vi "Function_Wizard.vi"(6 "Input":dbl[][](array[numeric]), 7 "Device References":refnum<vi>[](array[refnum]), 8 "Device properties":cluster{"Number of axes":i32}[](array[cluster]), 9 "Device parameters":variant[](array[variant]), 10 "Device order":i32[](array[numeric])=[0, 1], 11 "Device description":string[][](array[string])) -> (3 "Output":dbl[][](array[numeric]))   [LabVIEW 2015]
uses:
  <vilib>/gmath/NI_Gmath.lvlib
panel:
  in  "Cancel Button":bool
  in  "OK Button":bool
  in  "Ordering":u16(ring) items=["Raster", "Serpentine"]
  in  "Expression":string
  in  "Scan pattern":u16(ring) items=["Linear", "Exponential", "Logarithmic", "Quadratic", "Custom"]
  in  "Parameter table":string[][](table)
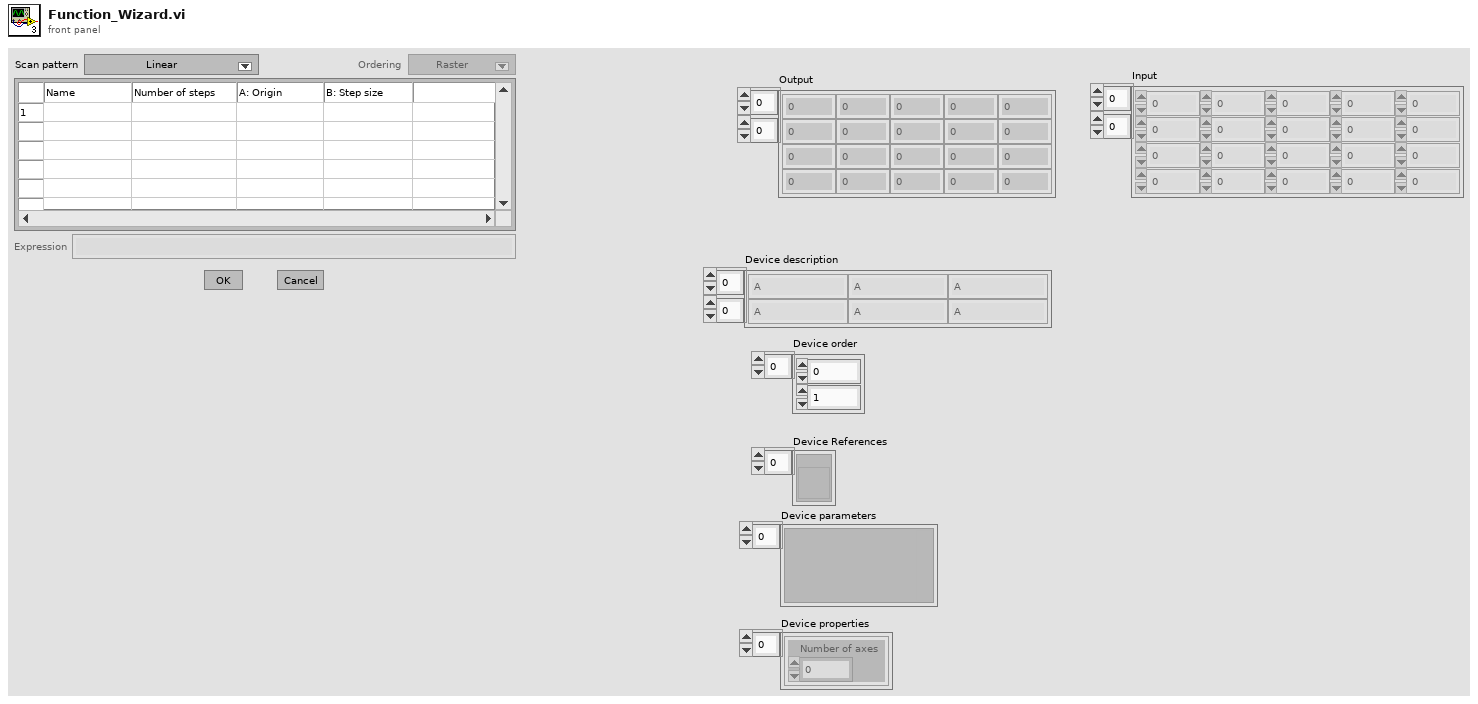
[diagram p1: front panel]
types:
  T1 = enum8{"Enabled", "Disabled", "Disabled and Grayed Out"}
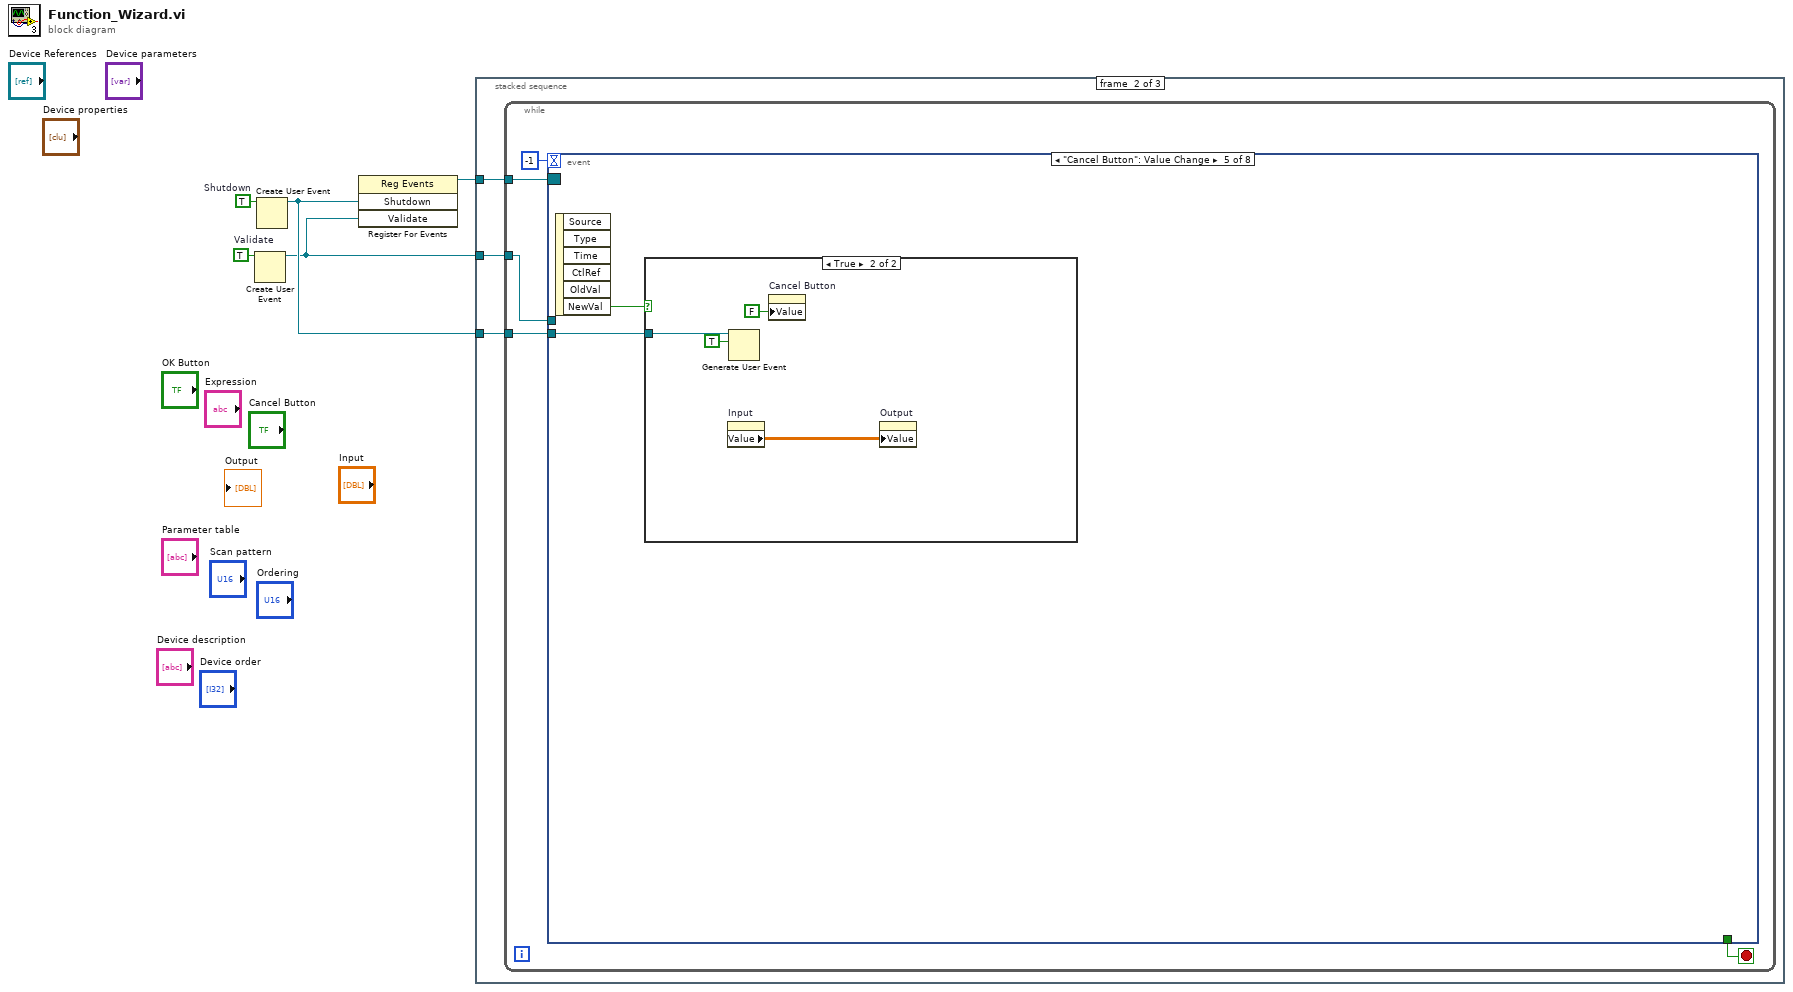
[diagram p0: block diagram]
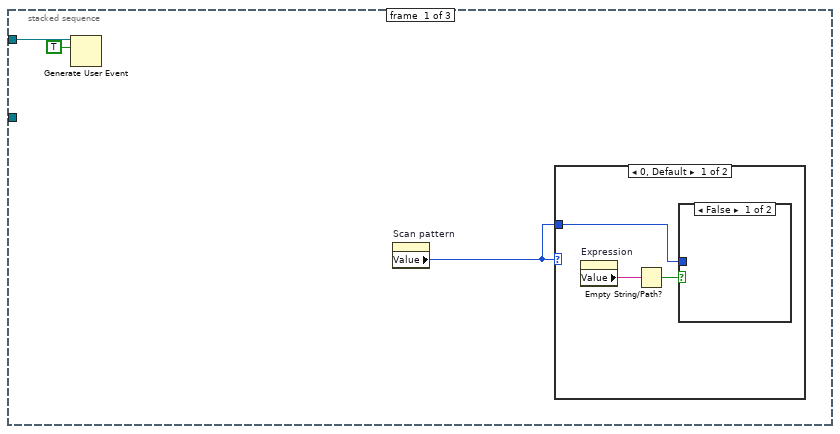
[diagram p2: hidden frame]
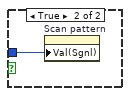
[diagram p3: hidden frame]
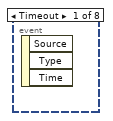
[diagram p5: hidden frame]
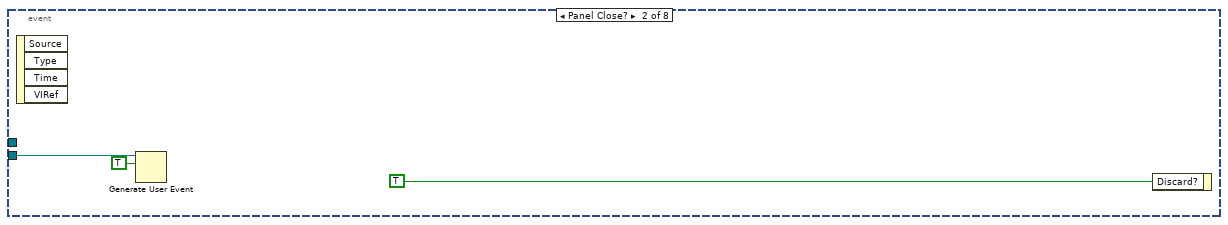
[diagram p6: hidden frame]
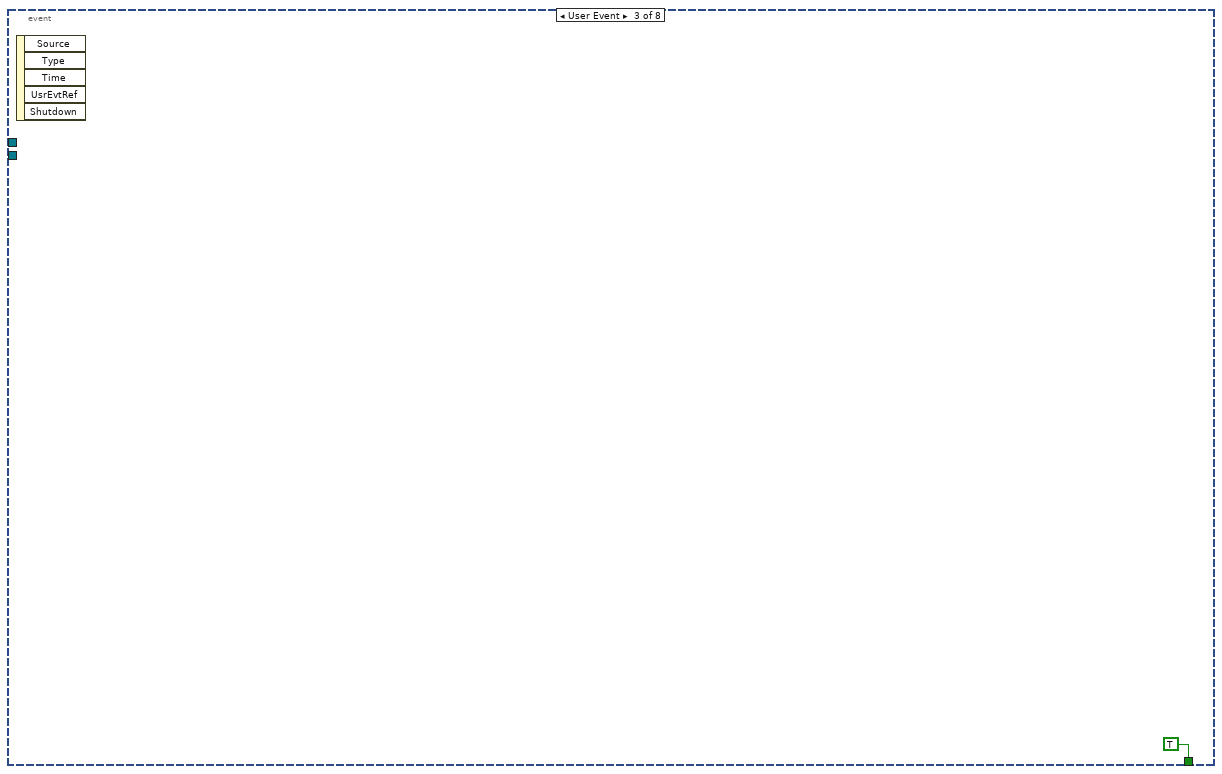
[diagram p7: hidden frame]
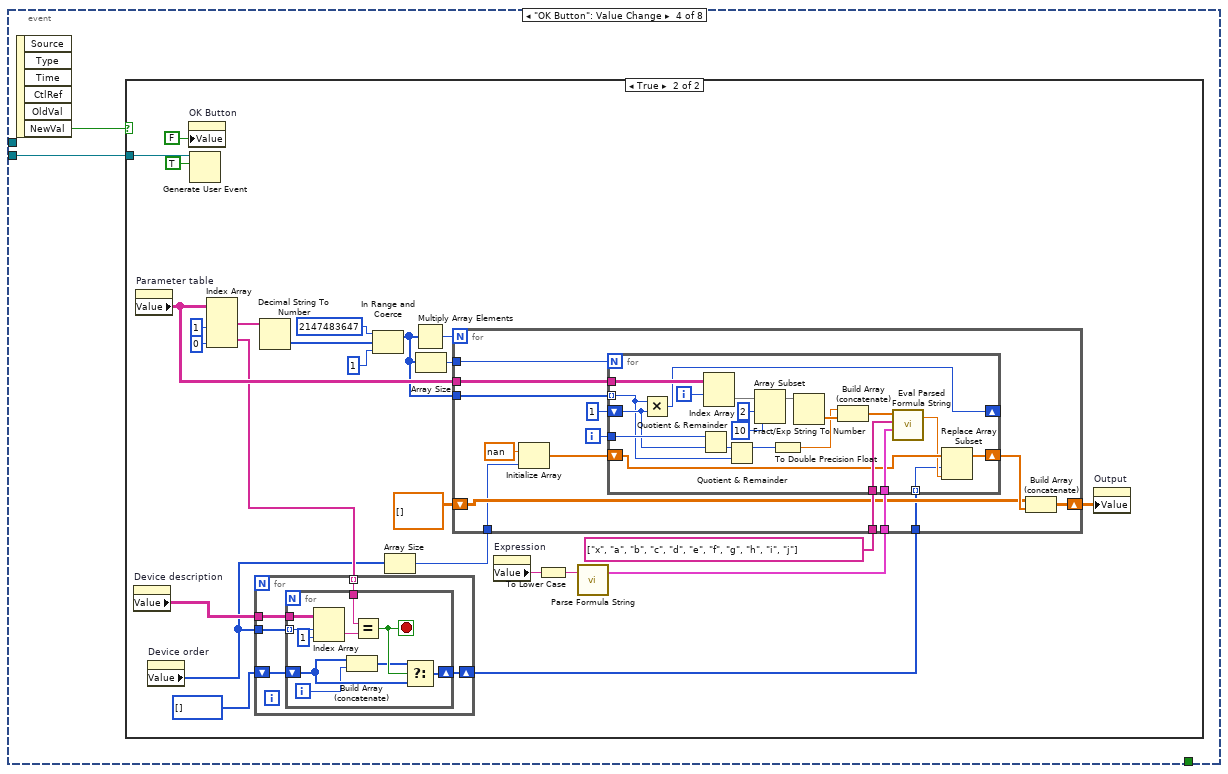
[diagram p8: hidden frame]
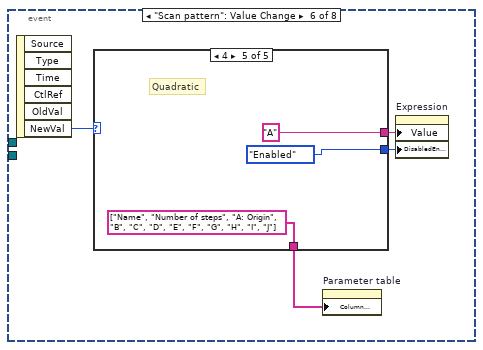
[diagram p11: hidden frame]
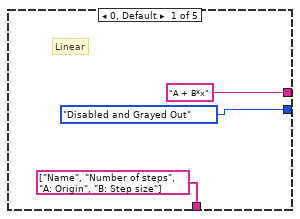
[diagram p12: hidden frame]
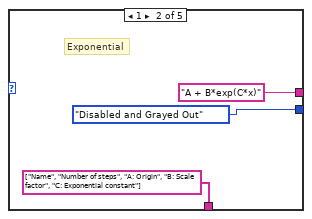
[diagram p13: hidden frame]
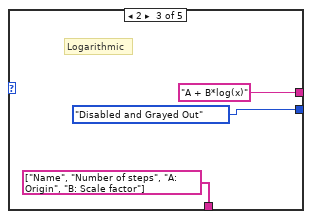
[diagram p14: hidden frame]
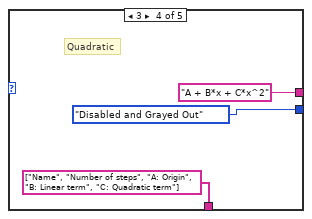
[diagram p15: hidden frame]
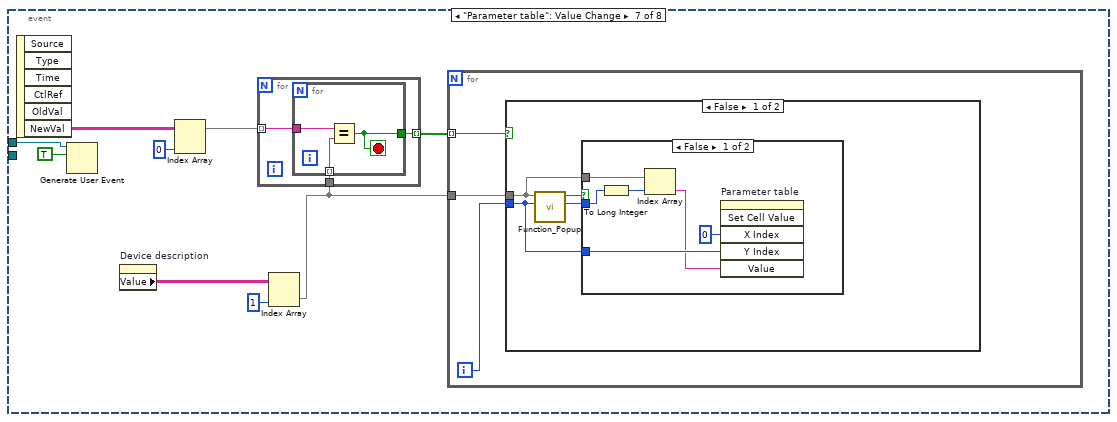
[diagram p16: hidden frame]
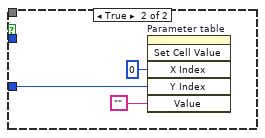
[diagram p17: hidden frame]
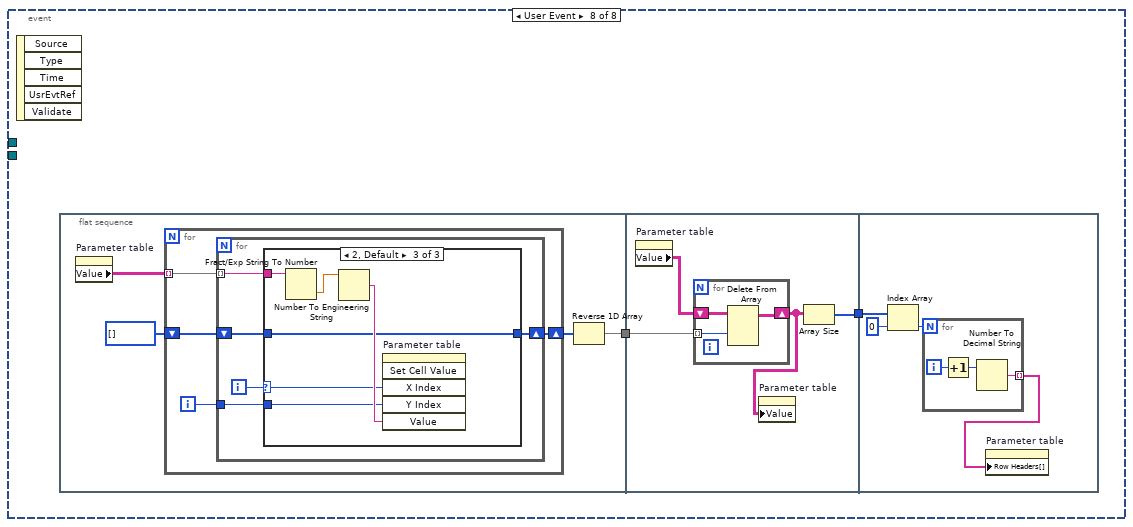
[diagram p19: hidden frame]
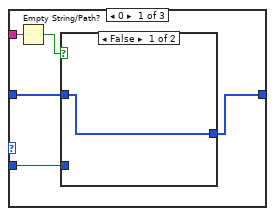
[diagram p20: hidden frame]
diagram:
  w2 = TRUE  # Validate
  w4 = TRUE  # Shutdown
  n1 = Create User Event(user event datatype=w2) -> (user event=w1:refnum<user-event>)  [unwired: 1 in, 1 out]
  n2 = Create User Event(user event datatype=w4) -> (user event=w3:refnum<user-event>)  [unwired: 1 in, 1 out]
  n3 = register-events(w3, w1) -> (reference out=w5:refnum<event-registration>)  [unwired: 2 in, 1 out]
  n4 = stacked-sequence {
    tunnel: w5 -> [_ w15 _]
    tunnel: w3 -> [_ w14 w208]
    tunnel: w1 -> [w8 w13 w209]
    frame #0 {
      n5 = Generate User Event(user event=w8, event data cluster=TRUE ("event data")) -> ()  [unwired: 2 in, 2 out]
      n6 = property on="Scan pattern" class="Ring (strict)"() -> ("Value"=w6:u16)  [unwired: 2 in, 2 out]
      n7 = case shown="0, Default" w6 {
        tunnel: w6 -> [w9 _]
        frame 0, Default {
          n8 = property on="Expression" class="Str"() -> ("Value"=w11:string)  [unwired: 2 in, 2 out]
          n9 = Empty String/Path?(string/path=w11) -> (empty?=w10:bool)
          n10 = case shown="False" w10 {
            tunnel: w9 -> [_ w12]
            frame False {
            }
            frame True {
              n11 = property on="Scan pattern" class="Ring (strict)"("Val(Sgnl)"=w12) -> ()  [unwired: 2 in, 2 out]
            }
          }
        }
        frame 4 {
        }
      }
    }
    frame #1 {
      n12 = while {
        tunnel: w15 -> [w19]
        tunnel: w14 -> [w17]
        tunnel: w13 -> [w16]
        stop <- w18 stop-if-true
        n13 = event shown="[4] \"Cancel Button\": Value Change" {
          selector: w19 -> [_ _ _ _ _ _ _ _]
          dyn-events: _ -> [_ _ _ _ _ _ _ _]
          timeout: -1 -> [_ _ _ _ _ _ _ _]
          tunnel: [_ _ TRUE _ _ _ _ _] -> w18
          tunnel: w17 -> [_ w22 _ w26 w103 _ _ _]
          tunnel: w16 -> [_ _ _ _ _ _ w135 _]
          event Timeout {
            n14 = event-data() -> ()  [unwired: 1 in, 3 out]
          }
          event Panel Close? {
            n15 = event-data() -> ()  [unwired: 1 in, 4 out]
            n16 = Generate User Event(user event=w22, event data cluster=TRUE ("event data")) -> ()  [unwired: 2 in, 2 out]
            n17 = event-data("Discard?"=TRUE) -> ()  [unwired: 1 in, 1 out]
          }
          event User Event {
            n18 = event-data() -> ()  [unwired: 1 in, 5 out]
          }
          event "OK Button": Value Change {
            n19 = event-data() -> ("NewVal"=w25:bool)  [unwired: 1 in, 5 out]
            n20 = case shown="True" w25 {
              tunnel: w26 -> [_ w51]
              frame False {
              }
              frame True {
                n21 = property on="Device description" class="Arr (strict)"() -> ("Value"=w32:string[][])  [unwired: 2 in, 2 out]
                n22 = property on="Parameter table" class="Tbl (strict)"() -> ("Value"=w41:string[][])  [unwired: 2 in, 2 out]
                n23 = property on="Device order" class="Arr (strict)"() -> ("Value"=w27:i32[])  [unwired: 2 in, 2 out]
                n24 = property on="OK Button" class="Bool (strict)"("Value"=FALSE ("OK Button")) -> ()  [unwired: 2 in, 2 out]
                n25 = Generate User Event(user event=w51, event data cluster=TRUE ("event data")) -> ()  [unwired: 2 in, 2 out]
                n26 = Index Array(array=w41, index (col) #1=1 ("disabled index (col)"), index (col) #2=0 ("index (col)")) -> (element #1=w47:string[], element #2=w31:string[])  [unwired: 2 in]
                n27 = for {
                  tunnel: w32 -> [w56]
                  tunnel: w27 -> [w55]
                  tunnel: w31 -> [w54] mode=indexing
                  shift-right: [w52] -> w29
                  shift-left: i32[] [] -> [w53]
                  n28 = for {
                    tunnel: w56 -> [w66]
                    tunnel: w55 -> [w65] mode=indexing
                    tunnel: w54 -> [w63]
                    shift-right: [w61] -> w52
                    shift-left: w53 -> [w60]
                    i -> [w57]
                    stop <- w62 stop-if-true
                    n29 = Index Array(array=w66, index (row)=w65, index (col)=1 ("disabled index (col)")) -> (element=w58:string)
                    n30 = Build Array (concatenate)(w60, w57) -> (w59:i32[])
                    n31 = Equal?(x=w63, y=w58) -> (x = y?=w62:bool)
                    n32 = Select(t=w59, s=w62, f=w60) -> (s? t:f=w61:i32[])
                  }
                }
                n33 = Decimal String To Number(string=w47) -> (number=w46:i32[])  [unwired: 2 in, 1 out]
                n34 = In Range and Coerce(upper limit=2147483647, x=w46, lower limit=1) -> (coerced(x)=w38:i32[])  [unwired: 1 out]
                n35 = Array Size(array=w27) -> (size(s)=w28:i32)
                n36 = Multiply Array Elements(1:w38) -> (0:w44:i32)
                n37 = Array Size(array=w38) -> (size(s)=w43:i32)
                n38 = property on="Expression" class="Str"() -> ("Value"=w35:string)  [unwired: 2 in, 2 out]
                n39 = To Lower Case(string=w35) -> (all lower case string=w34:string)
                n40 = call <vilib>:"Parse Formula String.vi"("formula"=w34) -> ("Parsed Formula"=w40:cluster{"Table":i32[][], "Y Values":dbl[]})  [unwired: 1 in, 1 out]
                n41 = for {
                  N: w44 -> [_]
                  tunnel: w43 -> [w78]
                  tunnel: w41 -> [w80]
                  tunnel: w40 -> [w76]
                  tunnel: string[] ["x", "a", "b", "c", "d", "e", "f", "g", "h", "i", "j"] ("Variables") -> [w75]
                  tunnel: w38 -> [w70]
                  shift-right: [w71] -> w36
                  shift-left: dbl[][] [] -> [w72]
                  tunnel: w29 -> [w68]
                  tunnel: w28 -> [w67]
                  i -> [w74]
                  n42 = Initialize Array(nan ("element"), w67) -> (w79:dbl[])
                  n43 = for {
                    N: w78 -> [_]
                    tunnel: w80 -> [w101]
                    shift-right: [w89] -> w73
                    shift-left: w79 -> [w88]
                    tunnel: w76 -> [w97]
                    tunnel: w75 -> [w96]
                    tunnel: w74 -> [w85]
                    shift-right: [w92] -> _
                    shift-left: 1 -> [w83]
                    tunnel: w70 -> [w82] mode=indexing
                    tunnel: w68 -> [w81] mode=indexing
                    i -> [w86]
                    n44 = Multiply(x=w82, y=w83) -> (x*y=w92:i32)
                    n45 = Quotient & Remainder(x=w85, y=w83) -> (floor(x/y)=w84:i32)  [unwired: 1 out]
                    n46 = Index Array(array=w101, index (row)=w86) -> (element=w100:string[])  [unwired: 1 in]
                    n47 = Quotient & Remainder(x=w84, y=w82) -> (x-y*floor(x/y)=w91:i32)  [unwired: 1 out]
                    n48 = Array Subset(array=w100, index=2, length=10) -> (w99:string[])
                    n49 = To Double Precision Float(number=w91) -> (double precision float=w90:dbl)
                    n50 = Fract/Exp String To Number(string=w99) -> (number=w95:dbl[])  [unwired: 3 in, 1 out]
                    n51 = Build Array (concatenate)(w90, w95) -> (w94:dbl[])
                    n52 = call <vilib>:"Eval Parsed Formula String.vi"("Parsed Formula"=w97, "Variables"=w96, "X Values"=w94) -> ("y value"=w87:dbl)  [unwired: 1 in, 1 out]
                    n53 = Replace Array Subset(array=w88, new element=w87, index=w81) -> (w89:dbl[])
                  }
                  n54 = Build Array (concatenate)(w72, w73) -> (w71:dbl[][])
                }
                n55 = property on="Output" class="Arr (strict)"("Value"=w36) -> ()  [unwired: 2 in, 2 out]
              }
            }
          }
          event "Cancel Button": Value Change {
            n56 = event-data() -> ("NewVal"=w102:bool)  [unwired: 1 in, 5 out]
            n57 = case shown="True" w102 {
              tunnel: w103 -> [_ w107]
              frame False {
              }
              frame True {
                n58 = property on="Input" class="Arr (strict)"() -> ("Value"=w104:dbl[][])  [unwired: 2 in, 2 out]
                n59 = Generate User Event(user event=w107, event data cluster=TRUE ("event data")) -> ()  [unwired: 2 in, 2 out]
                n60 = property on="Cancel Button" class="Bool (strict)"("Value"=FALSE ("Cancel Button")) -> ()  [unwired: 2 in, 2 out]
                n61 = property on="Output" class="Arr (strict)"("Value"=w104) -> ()  [unwired: 2 in, 2 out]
              }
            }
          }
          event "Scan pattern": Value Change {
            n62 = event-data() -> ("NewVal"=w111:u16)  [unwired: 1 in, 5 out]
            n63 = case shown="4" w111 {
              tunnel: ["A + B*x" "A + B*exp(C*x)" "A + B*log(x)" "A + B*x + C*x^2" "A"] -> w110
              tunnel: [T1."Disabled and Grayed Out" ("Disabled") T1."Disabled and Grayed Out" ("Disabled") T1."Disabled and Grayed Out" ("Disabled") T1."Disabled and Grayed Out" ("Disabled") T1."Enabled" ("Disabled")] -> w109
              tunnel: [string[] ["Name", "Number of steps", "A: Origin", "B: Step size"] ("Column Header Strings[]") string[] ["Name", "Number of steps", "A: Origin", "B: Scale factor", "C: Exponential constant"] ("Column Header Strings[]") string[] ["Name", "Number of steps", "A: Origin", "B: Scale factor"] ("Column Header Strings[]") string[] ["Name", "Number of steps", "A: Origin", "B: Linear term", "C: Quadratic term"] ("Column Header Strings[]") string[] ["Name", "Number of steps", "A: Origin", "B", "C", "D", "E", "F", "G", "H", "I", "J"] ("Column Header Strings[]")] -> w108
              frame 0, Default {
                # "Linear"
              }
              frame 1 {
                # "Exponential"
              }
              frame 2 {
                # "Logarithmic"
              }
              frame 3 {
                # "Quadratic"
              }
              frame 4 {
                # "Quadratic"
              }
            }
            n64 = property on="Parameter table" class="Tbl (strict)"("Column Headers[]"=w108) -> ()  [unwired: 2 in, 2 out]
            n65 = property on="Expression" class="Str"("Value"=w110, "DisabledEnum"=w109) -> ()  [unwired: 2 in, 2 out]
          }
          event "Parameter table": Value Change {
            n66 = event-data() -> ("NewVal"=w131:string[][])  [unwired: 1 in, 5 out]
            n67 = Generate User Event(user event=w135, event data cluster=TRUE ("event data")) -> ()  [unwired: 2 in, 2 out]
            n68 = property on="Device description" class="Arr (strict)"() -> ("Value"=w133:string[][])  [unwired: 2 in, 2 out]
            n69 = Index Array(array=w131, index (col)=0 ("disabled index (col)")) -> (element=w130:string[])  [unwired: 1 in]
            n70 = Index Array(array=w133, index (col)=1 ("disabled index (col)")) -> (element=w128:string[])  [unwired: 1 in]
            n71 = for {
              tunnel: w130 -> [w138] mode=indexing
              tunnel: w128 -> [w137]
              tunnel: [w136] -> w127 mode=indexing
              n72 = for {
                tunnel: w138 -> [w140]
                tunnel: w137 -> [w141] mode=indexing
                tunnel: [w139] -> w136
                stop <- w139 stop-if-true
                n73 = Equal?(x=w140, y=w141) -> (x = y?=w139:bool)
              }
            }
            n74 = for {
              tunnel: w127 -> [w144] mode=indexing
              tunnel: w128 -> [w142]
              i -> [w143]
              n75 = case shown="False" w144 {
                tunnel: w143 -> [w147 _]
                tunnel: w142 -> [w145 _]
                frame False {
                  n76 = call "Function_Popup.vi"("Row"=w147, "Axes"=w145) -> ("Selection"=w146:u16, "Cancelled"=w148:bool)  [unwired: 8 in]
                  n77 = case shown="False" w148 {
                    tunnel: w147 -> [w154 w157]
                    tunnel: w146 -> [w151 _]
                    tunnel: w145 -> [w152 _]
                    frame False {
                      n78 = To Long Integer(number=w151) -> (32bit integer=w149:i32)
                      n79 = Index Array(array=w152, index=w149) -> (element=w150:string)
                      n80 = invoke on="Parameter table" class="Tbl (strict)" method="Set Cell Value"("X Index"=0, "Y Index"=w154, "Value"=w150) -> ()  [unwired: 3 in, 6 out]
                    }
                    frame True {
                      n81 = invoke on="Parameter table" class="Tbl (strict)" method="Set Cell Value"("X Index"=0, "Y Index"=w157, "Value"="") -> ()  [unwired: 3 in, 6 out]
                    }
                  }
                }
                frame True {
                }
              }
            }
          }
          event User Event {
            n82 = event-data() -> ()  [unwired: 1 in, 5 out]
            n83 = flat-sequence {
              tunnel: [w162] -> w159
              tunnel: w159 -> [w197]
              tunnel: [w194] -> w158
              tunnel: w158 -> [w204]
              frame #0 {
                n84 = property on="Parameter table" class="Tbl (strict)"() -> ("Value"=w161:string[][])  [unwired: 2 in, 2 out]
                n85 = for {
                  tunnel: w161 -> [w167] mode=indexing
                  shift-right: [w165] -> w163
                  shift-left: i32[] [] -> [w164]
                  i -> [w166]
                  n86 = for {
                    tunnel: w167 -> [w171] mode=indexing
                    tunnel: w166 -> [w170]
                    shift-right: [w169] -> w165
                    shift-left: w164 -> [w168]
                    i -> [w172]
                    n87 = case shown="2, Default" w172 {
                      selector: w172 -> [_ w185 w192]
                      tunnel: w171 -> [w177 w183 w190]
                      tunnel: w170 -> [w175 w184 w191]
                      tunnel: [w174 w182 w188] -> w169
                      tunnel: w168 -> [w173 w182 w188]
                      frame 0 {
                        n88 = Empty String/Path?(string/path=w177) -> (empty?=w176:bool)
                        n89 = case shown="False" w176 {
                          tunnel: w175 -> [_ w181]
                          tunnel: [w178 w180] -> w174
                          tunnel: w173 -> [w178 w179]
                          frame False {
                          }
                          frame True {
                            n90 = Build Array (concatenate)(w179, w181) -> (w180:i32[])
                          }
                        }
                      }
                      frame 1 {
                        n91 = Decimal String To Number(string=w183) -> (number=w186:i32)  [unwired: 2 in, 1 out]
                        n92 = Number To Decimal String(number=w186) -> (decimal integer string=w187:string)  [unwired: 1 in]
                        n93 = invoke on="Parameter table" class="Tbl (strict)" method="Set Cell Value"("X Index"=w185, "Y Index"=w184, "Value"=w187) -> ()  [unwired: 3 in, 6 out]
                      }
                      frame 2, Default {
                        n94 = Fract/Exp String To Number(string=w190) -> (number=w189:dbl)  [unwired: 3 in, 1 out]
                        n95 = Number To Engineering String(4:w189) -> (0:w193:string)  [unwired: 3 in]
                        n96 = invoke on="Parameter table" class="Tbl (strict)" method="Set Cell Value"("X Index"=w192, "Y Index"=w191, "Value"=w193) -> ()  [unwired: 3 in, 6 out]
                      }
                    }
                  }
                }
                n97 = Reverse 1D Array(array=w163) -> (reversed array=w162:i32[])
              }
              frame #1 {
                n98 = property on="Parameter table" class="Tbl (strict)"() -> ("Value"=w196:string[][])  [unwired: 2 in, 2 out]
                n99 = for {
                  tunnel: w197 -> [w200] mode=indexing
                  shift-right: [w198] -> w195
                  shift-left: w196 -> [w199]
                  n100 = Delete From Array(array=w199, index (row)=w200) -> (array with subset deleted=w198:string[][])  [unwired: 2 in, 1 out]
                }
                n101 = property on="Parameter table" class="Tbl (strict)"("Value"=w195) -> ()  [unwired: 2 in, 2 out]
                n102 = Array Size(array=w195) -> (size(s)=w194:i32[])
              }
              frame #2 {
                n103 = Index Array(array=w204, index=0) -> (element=w202:i32)
                n104 = for {
                  N: w202 -> [_]
                  tunnel: [w206] -> w201 mode=indexing
                  i -> [w207]
                  n105 = Increment(x=w207) -> (x+1=w205:i32)
                  n106 = Number To Decimal String(number=w205) -> (decimal integer string=w206:string)  [unwired: 1 in]
                }
                n107 = property on="Parameter table" class="Tbl (strict)"("Row Headers[]"=w201) -> ()  [unwired: 2 in, 2 out]
              }
            }
          }
        }
      }
    }
    frame #2 {
      n108 = Destroy User Event(user event=w208) -> ()  [unwired: 1 in, 1 out]
      n109 = Destroy User Event(user event=w209) -> ()  [unwired: 1 in, 1 out]
    }
  }
